vi "Format LPC wavelength string to nm.vi"(8 "error in (no error)":errorcluster, 10 "String":string) -> (0 "error out":errorcluster, 2 "wavelength":dbl[unit])   [LabVIEW 2017]
doc: "Takes an input string from the LPC (laser power controller) and returns a wavelength reading in nm. If the string is formatted incorrectly or no wavelength is found, it returns -1 as the wavelength."
uses:
  <vilib>/Utility/error.llb/DialogType.ctl
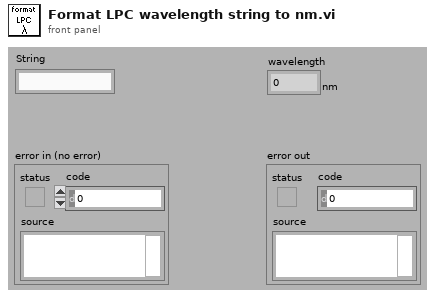
[diagram p1: front panel]
types:
  T1 = typedef "DialogType.ctl" = u16
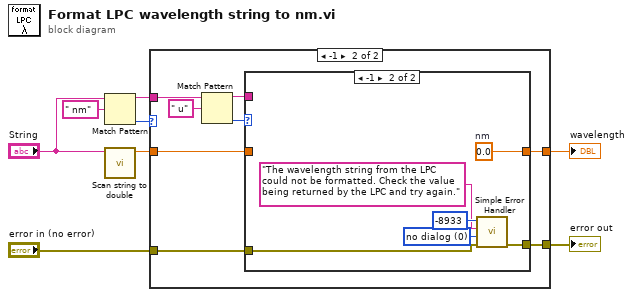
[diagram p0: block diagram]
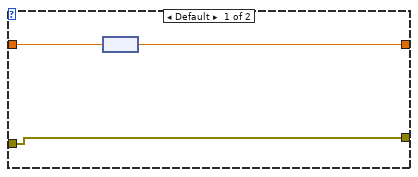
[diagram p2: hidden frame]
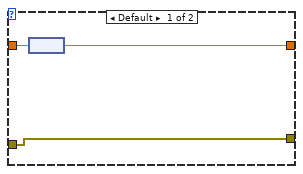
[diagram p3: hidden frame]
diagram:
  n1 = Match Pattern(string="String", regular expression=" nm") -> (before substring=w3:string, offset past match=w6:i32)  [unwired: 3 out]
  n2 = call "Scan string to double.vi"("String"="String") -> ("number"=w5:dbl)  [unwired: 1 in, 9 out]
  n3 = case shown="-1" w6 {
    tunnel: w5 -> [w11 w16]
    tunnel: [w10 w15] -> w4
    tunnel: w3 -> [_ w18]
    tunnel: "error in (no error)" -> [w9 w13]
    tunnel: [w9 w12] -> w1
    frame Default {
      n4 = node(w11) -> (w10:dbl[unit])
    }
    frame -1 {
      n5 = Match Pattern(string=w18, regular expression=" u") -> (before substring=w14:string, offset past match=w17:i32)  [unwired: 3 out]
      n6 = case shown="-1" w17 {
        tunnel: w16 -> [w21 _]
        tunnel: [w22 w28] -> w15
        tunnel: w14 -> [_ _]
        tunnel: w13 -> [w20 w24]
        tunnel: [w20 w23] -> w12
        frame Default {
          n7 = node(w21) -> (w22:dbl[unit])
        }
        frame -1 {
          w25 = T1 0 items=["no dialog", "OK message", "continue or stop message", "OK message + warnings", "continue/stop + warnings"] ("type of dialog (OK msg:1)")
          w28 = dbl[unit] 0.0  # nm
          n8 = call <vilib>:"Simple Error Handler.vi"("error code (no error:0)"=-8933, "error source (\" \")"="The wavelength string from the LPC could not be formatted. Check the value being returned by the LPC and try again." ("error source (\" \")"), "type of dialog (OK msg:1)"=w25, "error in (no error)"=w24) -> ("error out"=w23:errorcluster)  [unwired: 5 out]
        }
      }
    }
  }
  "wavelength" <- w4
  "error out" <- w1
